vi "Mask Write Register Request.vi"(7 "OR mask":u16, 8 "error in (no error)":errorcluster, 9 "AND mask":u16, 10 "starting address":u16) -> (0 "error out":errorcluster, 1 "Modbus Data Unit out":T1={"function"=1, "Data"=[]} {"function" items=["Read Discrete Inputs"=2, "Read Coils"=1, "Write Single Coil"=5, "Write Multiple Coils"=15, "Read Input Register"=4, "Read Holding Registers"=3, "Write Single Register"=6, "Write Multiple Registers"=16, "Read/Write Multiple Registers"=23, "Mask Write Register"=22, "Read FIFO Queue"=24, "Read File Record"=20, "Write File Record"=21, "Read Exception Status"=7, "Diagnostic"=8, "Get Com Event Counter"=11, "Get Com Event Log"=12, "Report Slave ID"=17, "Read Device Identification"=43]; "Data" format="%.0x"})   [LabVIEW 2019, in "NI_modbus_upd.lvlib"]
doc: "This VI forms a modbus data unit for masked writing of a single holding register."
uses:
  NI_modbus_upd.lvlib
  Ctl/MB Modbus Data Unit.ctl
  Modbus Data Unit (PDU)/Function.ctl
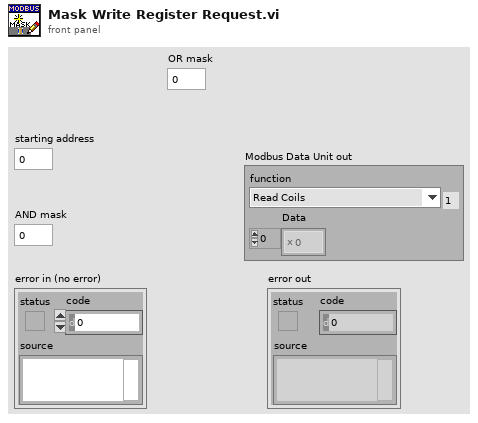
[diagram p1: front panel]
types:
  T1 = typedef "NI_modbus_upd.lvlib/MB Modbus Data Unit.ctl" = cluster{"function":T2, "Data":u8[]}
  T2 = typedef "NI_modbus_upd.lvlib/Function.ctl" = u8
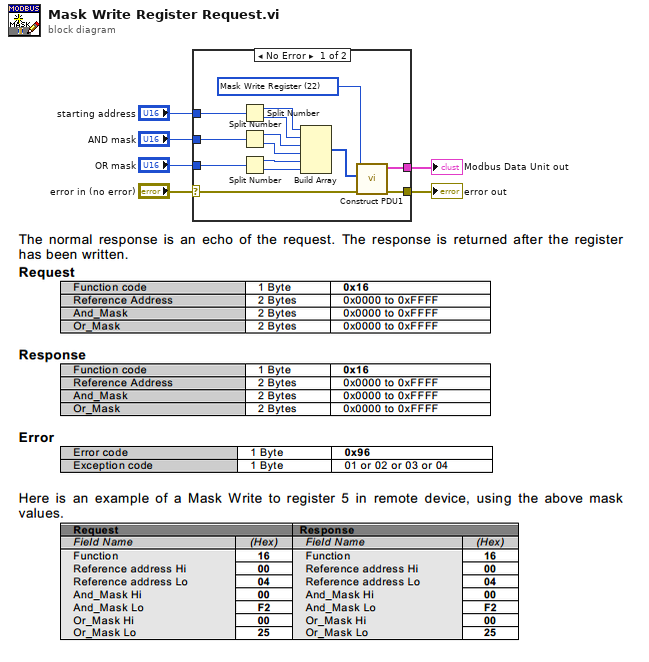
[diagram p0: block diagram]
diagram:
  n1 = case shown="No Error" "error in (no error)" {
    selector: "error in (no error)" -> [w7 w21]
    tunnel: [w20 w21] -> w6
    tunnel: "starting address" -> [w19 _]
    tunnel: [w18 _] -> w1
    tunnel: "AND mask" -> [w11 _]
    tunnel: "OR mask" -> [w10 _]
    frame No Error {
      w12 = T2 22 items=["Read Discrete Inputs"=2, "Read Coils"=1, "Write Single Coil"=5, "Write Multiple Coils"=15, "Read Input Register"=4, "Read Holding Registers"=3, "Write Single Register"=6, "Write Multiple Registers"=16, "Read/Write Multiple Registers"=23, "Mask Write Register"=22, "Read FIFO Queue"=24, "Read File Record"=20, "Write File Record"=21, "Read Exception Status"=7, "Diagnostic"=8, "Get Com Event Counter"=11, "Get Com Event Log"=12, "Report Slave ID"=17, "Read Device Identification"=43] ("Function")
      n2 = Split Number(x=w19) -> (hi(x)=w14:u8, lo(x)=w15:u8)
      n3 = Split Number(x=w11) -> (hi(x)=w16:u8, lo(x)=w17:u8)
      n4 = Split Number(x=w10) -> (hi(x)=w8:u8, lo(x)=w9:u8)
      n5 = Build Array(w14, w15, w16, w17, w8, w9) -> (w13:u8[])
      n6 = call "Construct PDU1.vi"("error in (no error)"=w7, "data"=w13, "function"=w12) -> ("error out"=w20:errorcluster, "Modbus Data Unit out"=w18:T1)  [unwired: 7 in]
    }
    frame Error {
    }
  }
  "error out" <- w6
  "Modbus Data Unit out" <- w1
